vi "Position Graph Legend Button.vi"(8 "error in (no error)":errorcluster, 10 "view legend":refnum<vi>, 11 "graph":refnum<vi>) -> (0 "error out":errorcluster)   [LabVIEW 2023, in "UI Helpers.lvlib"]
uses:
  UI Helpers.lvlib
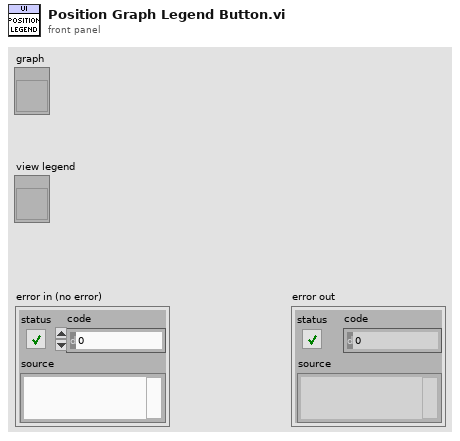
[diagram p1: front panel]
types:
  T1 = typedef "LVRectTypeDef.ctl" = cluster{"Left":i16, "Top":i16, "Right":i16, "Bottom":i16}
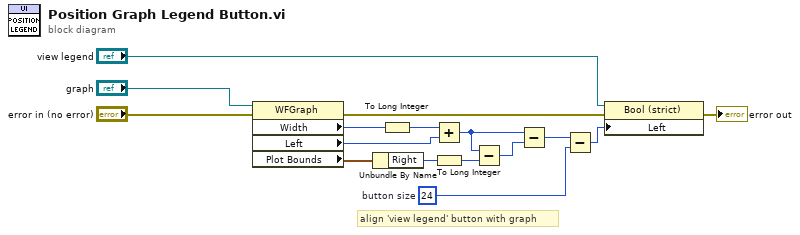
[diagram p0: block diagram]
diagram:
  w5 = 24  # button size
  # "align 'view legend' button with graph"
  n1 = property on="Property Node" class="WFGraph"(reference="graph", error in="error in (no error)") -> (error out=w2:errorcluster, "Width"=w11:u32, "Left"=w12:i32, "Plot Bounds"=w13:T1)  [unwired: 1 out]
  n2 = Unbundle By Name(w13) -> ("Right"=w4:i16)
  n3 = To Long Integer(number=w11) -> (32bit integer=w9:i32)
  n4 = Add(x=w9, y=w12) -> (x+y=w6:i32)
  n5 = To Long Integer(number=w4) -> (32bit integer=w10:i32)
  n6 = Subtract(x=w6, y=w10) -> (x-y=w7:i32)
  n7 = Subtract(x=w6, y=w7) -> (x-y=w8:i32)
  n8 = Subtract(x=w8, y=w5) -> (x-y=w14:i32)
  n9 = property on="Property Node" class="Bool (strict)"(reference="view legend", error in=w2, "Left"=w14) -> (error out=→"error out":errorcluster)  [unwired: 1 out]
